vi "updateSettings.vi"(8 "error in (no error)":errorcluster, 9 "ID":u32, 10 "Serial Number":string, 11 "Dosimetro in":refnum<class "Dosimetro.lvclass">) -> (0 "error out":errorcluster, 3 "Dosimetro out":refnum<class "Dosimetro.lvclass">)   [LabVIEW 2019, in "Dosimetro.lvclass"]
uses:
  Dosimetro.lvclass
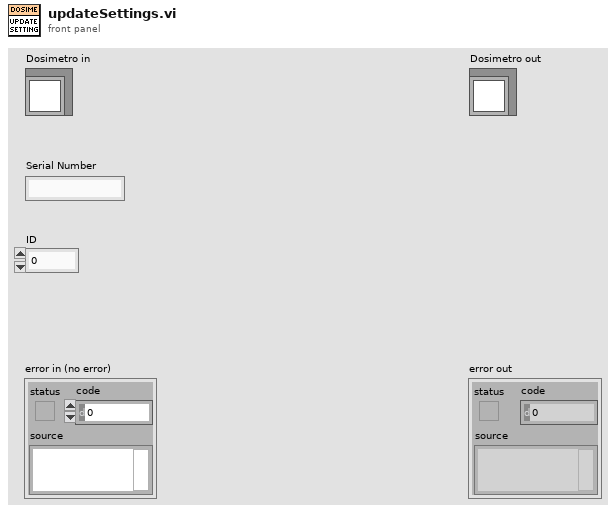
[diagram p1: front panel]
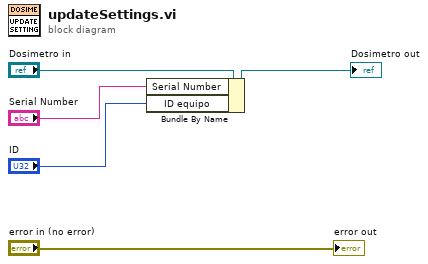
[diagram p0: block diagram]
diagram:
  n1 = Bundle By Name(cluster="Dosimetro in", "Serial Number"="Serial Number", "ID equipo"="ID") -> (→"Dosimetro out":refnum<class "Dosimetro.lvclass">)
  "error out" <- "error in (no error)"
